vi "car _ai.vi"() -> ()   [LabVIEW 2022 SP3]
uses:
  Control 1.ctl
  Control 2.ctl
  chicken.ctl
  plus_one.ctl
  game_over.ctl
panel:
  in  "v 10":dbl
  in  "v 9":dbl
  in  "v 8":dbl
  in  "v 7":dbl
  in  "v 6":dbl
  in  "v 5":dbl
  in  "v 4":dbl
  in  "v 3":dbl
  in  "v 2":dbl
  in  "v":dbl
  in  "state":i16
  in  "action":i16
  out "Boolean 12":T1
  in  "chicken":T2
  out "TOP":i16
  out "SCORE":i16
  in  "stop":bool
  out "Boolean 11":T3
  out "car_x":i16
  out "Boolean 10":T4
  out "Boolean 9":T5
  out "Boolean 8":T4
  out "Boolean 7":T5
  out "Boolean 6":T4
  out "Boolean 5":T5
  out "Boolean 4":T4
  out "Boolean 3":T5
  out "Boolean 2":T4
  out "Boolean":T5
  # "SCORE"
  # "TOP"
  # "Don't forget to reset the path of music first."
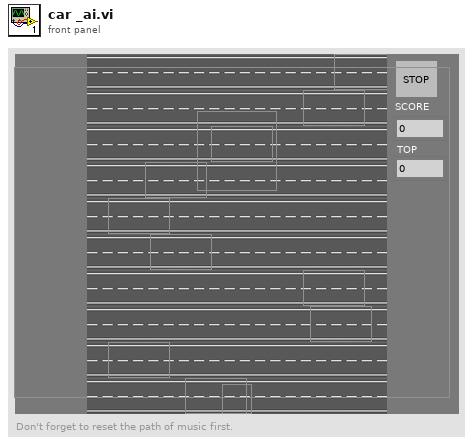
[diagram p1: front panel]
types:
  T1 = typedef "game_over.ctl" = bool
  T2 = typedef "chicken.ctl" = bool
  T3 = typedef "plus_one.ctl" = bool
  T4 = typedef "Control 2.ctl" = bool
  T5 = typedef "Control 1.ctl" = bool
  T6 = typedef "Sound Output Task ID.ctl" = u32
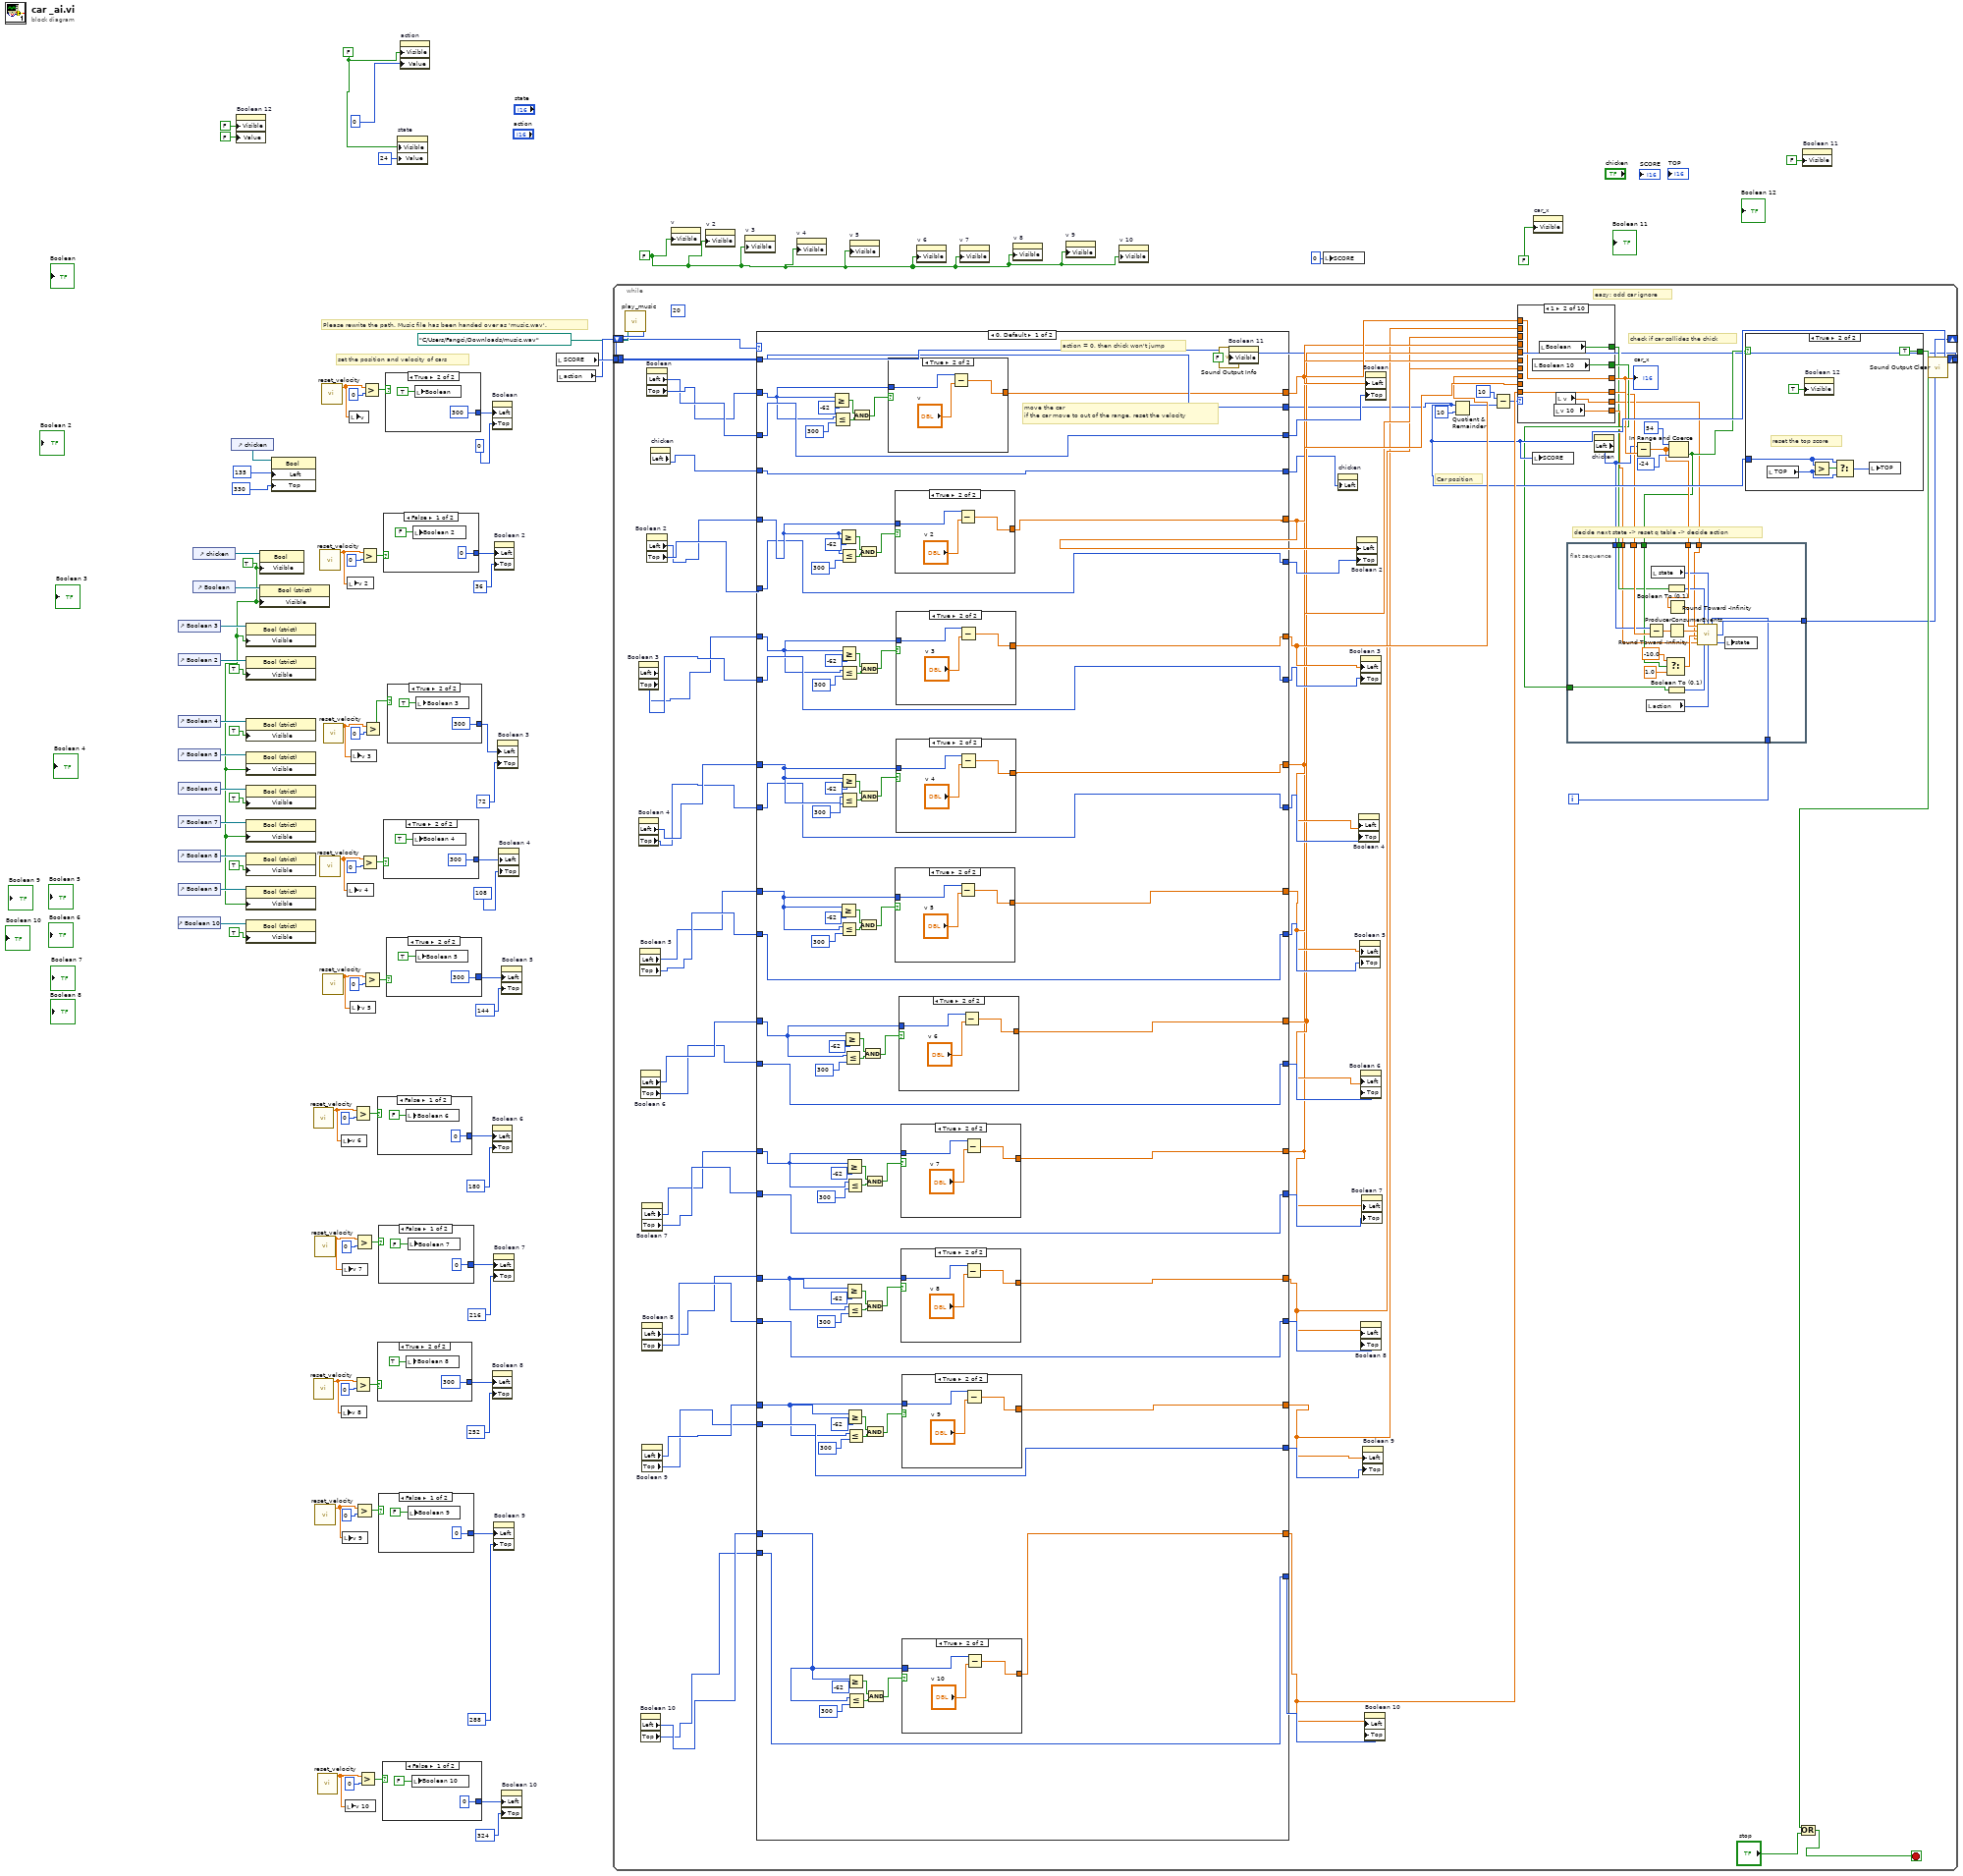
[diagram p0: block diagram]
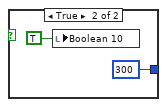
[diagram p2: hidden frame]
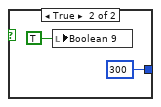
[diagram p3: hidden frame]
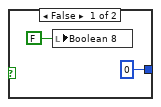
[diagram p4: hidden frame]
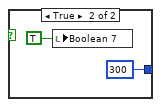
[diagram p5: hidden frame]
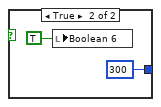
[diagram p6: hidden frame]
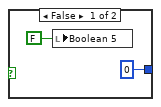
[diagram p7: hidden frame]
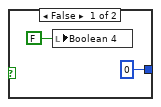
[diagram p8: hidden frame]
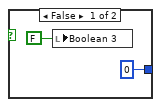
[diagram p9: hidden frame]
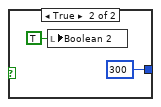
[diagram p10: hidden frame]
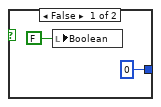
[diagram p11: hidden frame]
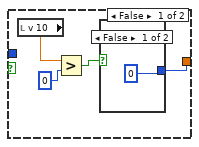
[diagram p12: hidden frame]
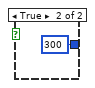
[diagram p13: hidden frame]
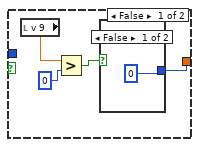
[diagram p14: hidden frame]
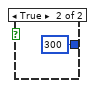
[diagram p15: hidden frame]
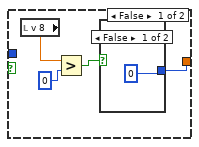
[diagram p16: hidden frame]
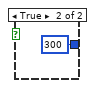
[diagram p17: hidden frame]
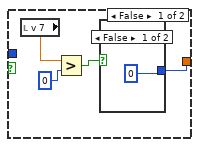
[diagram p18: hidden frame]
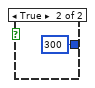
[diagram p19: hidden frame]
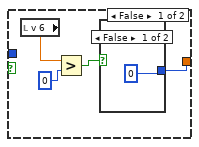
[diagram p20: hidden frame]
diagram:
  w19 = TRUE ("Visible")
  w14 = FALSE ("Visible")
  w17 = FALSE
  # "set the position and velocity of cars"
  # "Please rewrite the path. Music file has been handed over as 'music.wav'."
  n1 = control-ref of="Boolean 3"() -> (w27:refnum<vi>)
  n2 = control-ref of="Boolean 2"() -> (w28:refnum<vi>)
  n3 = control-ref of="Boolean 4"() -> (w29:refnum<vi>)
  n4 = control-ref of="Boolean 5"() -> (w30:refnum<vi>)
  n5 = control-ref of="Boolean 6"() -> (w31:refnum<vi>)
  n6 = control-ref of="Boolean 7"() -> (w32:refnum<vi>)
  n7 = control-ref of="Boolean 8"() -> (w33:refnum<vi>)
  n8 = control-ref of="Boolean 9"() -> (w34:refnum<vi>)
  n9 = control-ref of="Boolean 10"() -> (w36:refnum<vi>)
  n10 = control-ref of="chicken"() -> (w21:refnum<vi>)
  n11 = control-ref of="Boolean"() -> (w26:refnum<vi>)
  n12 = control-ref of="chicken"() -> (w41:refnum<vi>)
  n13 = property on="Boolean 12" class="Bool (strict)"("Visible"=FALSE, "Value"=T1 FALSE ("Boolean 12")) -> ()  [unwired: 2 in, 2 out]
  n14 = property class="Bool (strict)"(reference=w27, "Visible"=w19) -> ()  [unwired: 1 in, 2 out]
  n15 = property class="Bool (strict)"(reference=w28, "Visible"=TRUE) -> ()  [unwired: 1 in, 2 out]
  n16 = property class="Bool (strict)"(reference=w29, "Visible"=TRUE) -> ()  [unwired: 1 in, 2 out]
  n17 = property class="Bool (strict)"(reference=w30, "Visible"=w19) -> ()  [unwired: 1 in, 2 out]
  n18 = property class="Bool (strict)"(reference=w31, "Visible"=TRUE) -> ()  [unwired: 1 in, 2 out]
  n19 = property class="Bool (strict)"(reference=w32, "Visible"=w19) -> ()  [unwired: 1 in, 2 out]
  n20 = property class="Bool (strict)"(reference=w33, "Visible"=TRUE) -> ()  [unwired: 1 in, 2 out]
  n21 = property class="Bool (strict)"(reference=w34, "Visible"=w19) -> ()  [unwired: 1 in, 2 out]
  n22 = property class="Bool (strict)"(reference=w36, "Visible"=TRUE) -> ()  [unwired: 1 in, 2 out]
  n23 = property class="Bool"(reference=w21, "Visible"=w19) -> ()  [unwired: 1 in, 2 out]
  n24 = property class="Bool (strict)"(reference=w26, "Visible"=w19) -> ()  [unwired: 1 in, 2 out]
  n25 = property on="Property Node" class="Bool"(reference=w41, "Left"=135 ("Position:Left"), "Top"=330 ("Position:Top")) -> ()  [unwired: 1 in, 2 out]
  n26 = call "reset_velocity.vi"() -> ("Numeric"=w9:dbl)  [unwired: 11 in]
  n27 = call "reset_velocity.vi"() -> ("Numeric"=w11:dbl)  [unwired: 11 in]
  n28 = call "reset_velocity.vi"() -> ("Numeric"=w10:dbl)  [unwired: 11 in]
  n29 = call "reset_velocity.vi"() -> ("Numeric"=w12:dbl)  [unwired: 11 in]
  n30 = call "reset_velocity.vi"() -> ("Numeric"=w13:dbl)  [unwired: 11 in]
  n31 = call "reset_velocity.vi"() -> ("Numeric"=w5:dbl)  [unwired: 11 in]
  n32 = call "reset_velocity.vi"() -> ("Numeric"=w7:dbl)  [unwired: 11 in]
  n33 = call "reset_velocity.vi"() -> ("Numeric"=w4:dbl)  [unwired: 11 in]
  n34 = call "reset_velocity.vi"() -> ("Numeric"=w8:dbl)  [unwired: 11 in]
  n35 = call "reset_velocity.vi"() -> ("Numeric"=w6:dbl)  [unwired: 11 in]
  n36 = local write "v 6"(w9) -> ()
  n37 = local write "v 8"(w11) -> ()
  n38 = local write "v 7"(w10) -> ()
  n39 = local write "v 9"(w12) -> ()
  n40 = local write "v 10"(w13) -> ()
  n41 = local write "v 2"(w5) -> ()
  n42 = local write "v 4"(w7) -> ()
  n43 = local write "v"(w4) -> ()
  n44 = local write "v 5"(w8) -> ()
  n45 = local write "v 3"(w6) -> ()
  n46 = Greater?(x=w9, y=0) -> (0:w61:bool)
  n47 = Greater?(x=w11, y=0) -> (0:w53:bool)
  n48 = Greater?(x=w10, y=0) -> (0:w56:bool)
  n49 = Greater?(x=w12, y=0) -> (0:w48:bool)
  n50 = Greater?(x=w13, y=0) -> (0:w45:bool)
  n51 = Greater?(x=w5, y=0) -> (0:w77:bool)
  n52 = Greater?(x=w7, y=0) -> (0:w69:bool)
  n53 = Greater?(x=w4, y=0) -> (0:w80:bool)
  n54 = Greater?(x=w8, y=0) -> (0:w64:bool)
  n55 = Greater?(x=w6, y=0) -> (0:w72:bool)
  n56 = case shown="False" w61 {
    tunnel: [0 300] -> w59
    frame False {
      n57 = local write "Boolean 6"(FALSE) -> ()
    }
    frame True {
      n58 = local write "Boolean 6"(TRUE) -> ()
    }
  }
  n59 = case shown="True" w53 {
    tunnel: [0 300] -> w51
    frame False {
      n60 = local write "Boolean 8"(FALSE) -> ()
    }
    frame True {
      n61 = local write "Boolean 8"(TRUE) -> ()
    }
  }
  n62 = case shown="False" w56 {
    tunnel: [0 300] -> w55
    frame False {
      n63 = local write "Boolean 7"(FALSE) -> ()
    }
    frame True {
      n64 = local write "Boolean 7"(TRUE) -> ()
    }
  }
  n65 = case shown="False" w48 {
    tunnel: [0 300] -> w47
    frame False {
      n66 = local write "Boolean 9"(FALSE) -> ()
    }
    frame True {
      n67 = local write "Boolean 9"(TRUE) -> ()
    }
  }
  n68 = case shown="False" w45 {
    tunnel: [0 300] -> w43
    frame False {
      n69 = local write "Boolean 10"(FALSE) -> ()
    }
    frame True {
      n70 = local write "Boolean 10"(TRUE) -> ()
    }
  }
  n71 = case shown="False" w77 {
    tunnel: [0 300] -> w75
    frame False {
      n72 = local write "Boolean 2"(FALSE) -> ()
    }
    frame True {
      n73 = local write "Boolean 2"(TRUE) -> ()
    }
  }
  n74 = case shown="True" w69 {
    tunnel: [0 300] -> w67
    frame False {
      n75 = local write "Boolean 4"(FALSE) -> ()
    }
    frame True {
      n76 = local write "Boolean 4"(TRUE) -> ()
    }
  }
  n77 = case shown="True" w80 {
    tunnel: [0 300] -> w79
    frame False {
      n78 = local write "Boolean"(FALSE) -> ()
    }
    frame True {
      n79 = local write "Boolean"(TRUE) -> ()
    }
  }
  n80 = case shown="True" w64 {
    tunnel: [0 300] -> w63
    frame False {
      n81 = local write "Boolean 5"(FALSE) -> ()
    }
    frame True {
      n82 = local write "Boolean 5"(TRUE) -> ()
    }
  }
  n83 = case shown="True" w72 {
    tunnel: [0 300] -> w70
    frame False {
      n84 = local write "Boolean 3"(FALSE) -> ()
    }
    frame True {
      n85 = local write "Boolean 3"(TRUE) -> ()
    }
  }
  n86 = property on="state" class="DigNum (strict)"("Visible"=w17, "Value"=i16 24 ("state")) -> ()  [unwired: 2 in, 2 out]
  n87 = property on="action" class="DigNum (strict)"("Visible"=w17, "Value"=i16 0 ("done")) -> ()  [unwired: 2 in, 2 out]
  n88 = property on="Boolean" class="Bool (strict)"("Left"=w79, "Top"=0) -> ()  [unwired: 2 in, 2 out]
  n89 = property on="Boolean 6" class="Bool (strict)"("Left"=w59, "Top"=180) -> ()  [unwired: 2 in, 2 out]
  n90 = property on="Boolean 8" class="Bool (strict)"("Left"=w51, "Top"=252) -> ()  [unwired: 2 in, 2 out]
  n91 = property on="Boolean 7" class="Bool (strict)"("Left"=w55, "Top"=216) -> ()  [unwired: 2 in, 2 out]
  n92 = property on="Boolean 9" class="Bool (strict)"("Left"=w47, "Top"=288) -> ()  [unwired: 2 in, 2 out]
  n93 = property on="Boolean 2" class="Bool (strict)"("Left"=w75, "Top"=36) -> ()  [unwired: 2 in, 2 out]
  n94 = property on="Boolean 3" class="Bool (strict)"("Left"=w70, "Top"=72) -> ()  [unwired: 2 in, 2 out]
  n95 = property on="Boolean 4" class="Bool (strict)"("Left"=w67, "Top"=108) -> ()  [unwired: 2 in, 2 out]
  n96 = property on="Boolean 5" class="Bool (strict)"("Left"=w63, "Top"=144) -> ()  [unwired: 2 in, 2 out]
  n97 = property on="Boolean 10" class="Bool (strict)"("Left"=w43, "Top"=324) -> ()  [unwired: 2 in, 2 out]
  n98 = local read "SCORE"() -> (w20:i16)
  n99 = local read "action"() -> (w18:i16)
  n100 = call "play_music.vi"("Sound File Path"=path "C:/Users/Fangci/Downloads/music.wav") -> ("task ID"=w3:T6)  [unwired: 10 in]
  n101 = while {
    shift-right: [w140] -> _
    shift-left: w20 -> [w141]
    shift-right: [w129] -> _
    shift-left: w18 -> [w138]
    tunnel: w3 -> [w126]
    tunnel: [w125] -> w2
    i -> [w128]
    stop <- w127 stop-if-true
    (unwired) 20
    # "decide next state -> reset q table -> decide action"
    # "check if car collides the chick"
    # "easy: odd car ignore"
    # "Car position"
    n102 = property on="Boolean 3" class="Bool (strict)"() -> ("Left"=w184:i32, "Top"=w185:i32)  [unwired: 2 in, 2 out]
    n103 = property on="Boolean 4" class="Bool (strict)"() -> ("Left"=w182:i32, "Top"=w181:i32)  [unwired: 2 in, 2 out]
    n104 = property on="Boolean 5" class="Bool (strict)"() -> ("Left"=w171:i32, "Top"=w179:i32)  [unwired: 2 in, 2 out]
    n105 = property on="Boolean 6" class="Bool (strict)"() -> ("Left"=w177:i32, "Top"=w176:i32)  [unwired: 2 in, 2 out]
    n106 = property on="Boolean 10" class="Bool (strict)"() -> ("Left"=w164:i32, "Top"=w163:i32)  [unwired: 2 in, 2 out]
    n107 = property on="Boolean 7" class="Bool (strict)"() -> ("Left"=w170:i32, "Top"=w174:i32)  [unwired: 2 in, 2 out]
    n108 = property on="Boolean 8" class="Bool (strict)"() -> ("Left"=w169:i32, "Top"=w172:i32)  [unwired: 2 in, 2 out]
    n109 = property on="Boolean 9" class="Bool (strict)"() -> ("Left"=w167:i32, "Top"=w166:i32)  [unwired: 2 in, 2 out]
    n110 = property on="Boolean" class="Bool (strict)"() -> ("Left"=w190:i32, "Top"=w191:i32)  [unwired: 2 in, 2 out]
    n111 = property on="Boolean 2" class="Bool (strict)"() -> ("Left"=w188:i32, "Top"=w189:i32)  [unwired: 2 in, 2 out]
    n112 = property on="chicken" class="Bool"() -> ("Left"=w143:i32)  [unwired: 2 in, 2 out]
    n113 = case shown="0, Default" w138 {
      tunnel: [w223 w426] -> w186
      tunnel: w191 -> [w223 w425]
      tunnel: [w220 w424] -> w160
      tunnel: w190 -> [w222 w423]
      tunnel: [w217 w419] -> w187
      tunnel: w189 -> [w217 w420]
      tunnel: [w216 w421] -> w159
      tunnel: w188 -> [w218 w422]
      tunnel: [w214 w413] -> w183
      tunnel: w185 -> [w214 w414]
      tunnel: [w215 w415] -> w158
      tunnel: w184 -> [w213 w416]
      tunnel: [w211 w408] -> w180
      tunnel: w181 -> [w211 w407]
      tunnel: [w210 w406] -> w157
      tunnel: w182 -> [w212 w405]
      tunnel: [w208 w401] -> w178
      tunnel: w179 -> [w208 w402]
      tunnel: [w209 w403] -> w156
      tunnel: w171 -> [w207 w404]
      tunnel: [w206 w396] -> w175
      tunnel: w176 -> [w206 w395]
      tunnel: [w205 w394] -> w155
      tunnel: w177 -> [w204 w393]
      tunnel: [w202 w389] -> w173
      tunnel: w174 -> [w202 w390]
      tunnel: [w201 w391] -> w154
      tunnel: w170 -> [w203 w392]
      tunnel: [w199 w384] -> w168
      tunnel: w172 -> [w199 w383]
      tunnel: [w198 w382] -> w153
      tunnel: w169 -> [w200 w381]
      tunnel: [w196 w377] -> w165
      tunnel: w166 -> [w196 w378]
      tunnel: [w197 w379] -> w152
      tunnel: w167 -> [w195 w380]
      tunnel: [w192 w372] -> w162
      tunnel: w163 -> [w192 w371]
      tunnel: [w193 w370] -> w151
      tunnel: w164 -> [w194 w369]
      tunnel: w143 -> [w219 w367]
      tunnel: [w219 w367] -> w142
      tunnel: w141 -> [w221 w366]
      tunnel: [w221 w365] -> w140
      frame 0, Default {
        # "move the car\nif the car move to out of the range, reset the velocity"
        # "action = 0, then chick won't jump"
        n114 = Greater Or Equal?(x=w222, y=-62) -> (x >= y?=w246:bool)
        n115 = Less Or Equal?(x=w222, y=300) -> (x <= y?=w245:bool)
        n116 = Greater Or Equal?(x=w218, y=-62) -> (x >= y?=w249:bool)
        n117 = Greater Or Equal?(x=w207, y=-62) -> (x >= y?=w258:bool)
        n118 = Less Or Equal?(x=w218, y=300) -> (x <= y?=w250:bool)
        n119 = Greater Or Equal?(x=w213, y=-62) -> (x >= y?=w252:bool)
        n120 = Greater Or Equal?(x=w212, y=-62) -> (x >= y?=w255:bool)
        n121 = Less Or Equal?(x=w207, y=300) -> (x <= y?=w259:bool)
        n122 = Less Or Equal?(x=w213, y=300) -> (x <= y?=w253:bool)
        n123 = Less Or Equal?(x=w212, y=300) -> (x <= y?=w254:bool)
        n124 = Greater Or Equal?(x=w204, y=-62) -> (x >= y?=w261:bool)
        n125 = Less Or Equal?(x=w204, y=300) -> (x <= y?=w260:bool)
        n126 = Greater Or Equal?(x=w203, y=-62) -> (x >= y?=w264:bool)
        n127 = Greater Or Equal?(x=w200, y=-62) -> (x >= y?=w267:bool)
        n128 = Less Or Equal?(x=w203, y=300) -> (x <= y?=w265:bool)
        n129 = Less Or Equal?(x=w200, y=300) -> (x <= y?=w266:bool)
        n130 = Greater Or Equal?(x=w195, y=-62) -> (x >= y?=w270:bool)
        n131 = Less Or Equal?(x=w195, y=300) -> (x <= y?=w271:bool)
        n132 = Greater Or Equal?(x=w194, y=-62) -> (x >= y?=w273:bool)
        n133 = Less Or Equal?(x=w194, y=300) -> (x <= y?=w272:bool)
        n134 = And(x=w246, y=w245) -> (x .and. y?=w247:bool)
        n135 = And(x=w249, y=w250) -> (x .and. y?=w248:bool)
        n136 = And(x=w258, y=w259) -> (x .and. y?=w257:bool)
        n137 = And(x=w252, y=w253) -> (x .and. y?=w251:bool)
        n138 = And(x=w255, y=w254) -> (x .and. y?=w256:bool)
        n139 = And(x=w261, y=w260) -> (x .and. y?=w262:bool)
        n140 = And(x=w264, y=w265) -> (x .and. y?=w263:bool)
        n141 = And(x=w267, y=w266) -> (x .and. y?=w268:bool)
        n142 = And(x=w270, y=w271) -> (x .and. y?=w269:bool)
        n143 = And(x=w273, y=w272) -> (x .and. y?=w274:bool)
        n144 = case shown="True" w247 {
          tunnel: [w356 w363] -> w220
          tunnel: w222 -> [_ w362]
          frame False {
            n145 = local read "v"() -> (w359:dbl)
            n146 = Greater?(x=w359, y=0) -> (0:w357:bool)
            n147 = case shown="False" w357 {
              tunnel: [0 300] -> w356
              frame False {
              }
              frame True {
              }
            }
          }
          frame True {
            n148 = Subtract(x=w362, y="v") -> (x-y=w363:dbl)
          }
        }
        n149 = case shown="True" w248 {
          tunnel: [w347 w354] -> w216
          tunnel: w218 -> [_ w353]
          frame False {
            n150 = local read "v 2"() -> (w350:dbl)
            n151 = Greater?(x=w350, y=0) -> (0:w348:bool)
            n152 = case shown="False" w348 {
              tunnel: [0 300] -> w347
              frame False {
              }
              frame True {
              }
            }
          }
          frame True {
            n153 = Subtract(x=w353, y="v 2") -> (x-y=w354:dbl)
          }
        }
        n154 = case shown="True" w257 {
          tunnel: [w320 w327] -> w209
          tunnel: w207 -> [_ w326]
          frame False {
            n155 = local read "v 5"() -> (w323:dbl)
            n156 = Greater?(x=w323, y=0) -> (0:w321:bool)
            n157 = case shown="False" w321 {
              tunnel: [0 300] -> w320
              frame False {
              }
              frame True {
              }
            }
          }
          frame True {
            n158 = Subtract(x=w326, y="v 5") -> (x-y=w327:dbl)
          }
        }
        n159 = case shown="True" w251 {
          tunnel: [w338 w345] -> w215
          tunnel: w213 -> [_ w344]
          frame False {
            n160 = local read "v 3"() -> (w341:dbl)
            n161 = Greater?(x=w341, y=0) -> (0:w339:bool)
            n162 = case shown="False" w339 {
              tunnel: [0 300] -> w338
              frame False {
              }
              frame True {
              }
            }
          }
          frame True {
            n163 = Subtract(x=w344, y="v 3") -> (x-y=w345:dbl)
          }
        }
        n164 = case shown="True" w256 {
          tunnel: [w329 w336] -> w210
          tunnel: w212 -> [_ w335]
          frame False {
            n165 = local read "v 4"() -> (w332:dbl)
            n166 = Greater?(x=w332, y=0) -> (0:w330:bool)
            n167 = case shown="False" w330 {
              tunnel: [0 300] -> w329
              frame False {
              }
              frame True {
              }
            }
          }
          frame True {
            n168 = Subtract(x=w335, y="v 4") -> (x-y=w336:dbl)
          }
        }
        n169 = case shown="True" w262 {
          tunnel: [w311 w318] -> w205
          tunnel: w204 -> [_ w317]
          frame False {
            n170 = local read "v 6"() -> (w314:dbl)
            n171 = Greater?(x=w314, y=0) -> (0:w312:bool)
            n172 = case shown="False" w312 {
              tunnel: [0 300] -> w311
              frame False {
              }
              frame True {
              }
            }
          }
          frame True {
            n173 = Subtract(x=w317, y="v 6") -> (x-y=w318:dbl)
          }
        }
        n174 = case shown="True" w263 {
          tunnel: [w302 w309] -> w201
          tunnel: w203 -> [_ w308]
          frame False {
            n175 = local read "v 7"() -> (w305:dbl)
            n176 = Greater?(x=w305, y=0) -> (0:w303:bool)
            n177 = case shown="False" w303 {
              tunnel: [0 300] -> w302
              frame False {
              }
              frame True {
              }
            }
          }
          frame True {
            n178 = Subtract(x=w308, y="v 7") -> (x-y=w309:dbl)
          }
        }
        n179 = case shown="True" w268 {
          tunnel: [w293 w300] -> w198
          tunnel: w200 -> [_ w299]
          frame False {
            n180 = local read "v 8"() -> (w296:dbl)
            n181 = Greater?(x=w296, y=0) -> (0:w294:bool)
            n182 = case shown="False" w294 {
              tunnel: [0 300] -> w293
              frame False {
              }
              frame True {
              }
            }
          }
          frame True {
            n183 = Subtract(x=w299, y="v 8") -> (x-y=w300:dbl)
          }
        }
        n184 = case shown="True" w269 {
          tunnel: [w284 w291] -> w197
          tunnel: w195 -> [_ w290]
          frame False {
            n185 = local read "v 9"() -> (w287:dbl)
            n186 = Greater?(x=w287, y=0) -> (0:w285:bool)
            n187 = case shown="False" w285 {
              tunnel: [0 300] -> w284
              frame False {
              }
              frame True {
              }
            }
          }
          frame True {
            n188 = Subtract(x=w290, y="v 9") -> (x-y=w291:dbl)
          }
        }
        n189 = case shown="True" w274 {
          tunnel: [w275 w282] -> w193
          tunnel: w194 -> [_ w281]
          frame False {
            n190 = local read "v 10"() -> (w278:dbl)
            n191 = Greater?(x=w278, y=0) -> (0:w276:bool)
            n192 = case shown="False" w276 {
              tunnel: [0 300] -> w275
              frame False {
              }
              frame True {
              }
            }
          }
          frame True {
            n193 = Subtract(x=w281, y="v 10") -> (x-y=w282:dbl)
          }
        }
        n194 = property on="Boolean 11" class="Bool (strict)"("Visible"=FALSE) -> ()  [unwired: 2 in, 2 out]
      }
      frame 1 {
        # "move the car\nif the car move to out of the range, reset the velocity"
        # "action = 1, then chick  jumps"
        n195 = Less?(x=w420, y=324) -> (x < y?=w417:bool)
        n196 = Less?(x=w383, y=324) -> (x < y?=w386:bool)
        n197 = Less?(x=w414, y=324) -> (x < y?=w411:bool)
        n198 = Less?(x=w390, y=324) -> (x < y?=w387:bool)
        n199 = Less?(x=w371, y=324) -> (x < y?=w374:bool)
        n200 = Less?(x=w407, y=324) -> (x < y?=w410:bool)
        n201 = Less?(x=w402, y=324) -> (x < y?=w399:bool)
        n202 = Less?(x=w395, y=324) -> (x < y?=w398:bool)
        n203 = Less?(x=w378, y=324) -> (x < y?=w375:bool)
        n204 = Less?(x=w425, y=324) -> (x < y?=w428:bool)
        n205 = case shown="False" w417 {
          tunnel: [0 w563] -> w419
          tunnel: w420 -> [_ w562]
          tunnel: [w550 w560] -> w421
          tunnel: w422 -> [_ w559]
          frame False {
            n206 = call "reset_velocity.vi"() -> ("Numeric"=w549:dbl)  [unwired: 11 in]
            n207 = local write "v 2"(w549) -> ()
            n208 = Greater?(x=w549, y=0) -> (0:w554:bool)
            n209 = case shown="False" w554 {
              frame False {
                n210 = local write "Boolean 2"(FALSE) -> ()
              }
              frame True {
                n211 = local write "Boolean 2"(TRUE) -> ()
              }
            }
            n212 = Random Number (0-1)() -> (number: 0 to 1=w552:dbl)
            n213 = Multiply(x=w552, y=300) -> (x*y=w550:dbl)
          }
          frame True {
            n214 = Add(x=w562, y=36) -> (x+y=w563:i32)
            n215 = local read "v 2"() -> (w558:dbl)
            n216 = Subtract(x=w559, y=w558) -> (x-y=w560:dbl)
          }
        }
        n217 = case shown="False" w386 {
          tunnel: [0 w473] -> w384
          tunnel: w383 -> [_ w472]
          tunnel: [w460 w469] -> w382
          tunnel: w381 -> [_ w470]
          frame False {
            n218 = call "reset_velocity.vi"() -> ("Numeric"=w459:dbl)  [unwired: 11 in]
            n219 = local write "v 8"(w459) -> ()
            n220 = Greater?(x=w459, y=0) -> (0:w464:bool)
            n221 = case shown="False" w464 {
              frame False {
                n222 = local write "Boolean 8"(FALSE) -> ()
              }
              frame True {
                (unwired) 300
                n223 = local write "Boolean 8"(TRUE) -> ()
              }
            }
            n224 = Random Number (0-1)() -> (number: 0 to 1=w461:dbl)
            n225 = Multiply(x=w461, y=300) -> (x*y=w460:dbl)
          }
          frame True {
            n226 = Add(x=w472, y=36) -> (x+y=w473:i32)
            n227 = local read "v 8"() -> (w468:dbl)
            n228 = Subtract(x=w470, y=w468) -> (x-y=w469:dbl)
          }
        }
        n229 = case shown="False" w411 {
          tunnel: [0 w548] -> w413
          tunnel: w414 -> [_ w547]
          tunnel: [w535 w544] -> w415
          tunnel: w416 -> [_ w545]
          frame False {
            n230 = call "reset_velocity.vi"() -> ("Numeric"=w534:dbl)  [unwired: 11 in]
            n231 = local write "v 3"(w534) -> ()
            n232 = Greater?(x=w534, y=0) -> (0:w539:bool)
            n233 = case shown="True" w539 {
              frame False {
                (unwired) 0
                n234 = local write "Boolean 3"(FALSE) -> ()
              }
              frame True {
                n235 = local write "Boolean 3"(TRUE) -> ()
              }
            }
            n236 = Random Number (0-1)() -> (number: 0 to 1=w537:dbl)
            n237 = Multiply(x=w537, y=300) -> (x*y=w535:dbl)
          }
          frame True {
            n238 = Add(x=w547, y=36) -> (x+y=w548:i32)
            n239 = local read "v 3"() -> (w543:dbl)
            n240 = Subtract(x=w545, y=w543) -> (x-y=w544:dbl)
          }
        }
        n241 = case shown="False" w387 {
          tunnel: [0 w488] -> w389
          tunnel: w390 -> [_ w487]
          tunnel: [w475 w484] -> w391
          tunnel: w392 -> [_ w485]
          frame False {
            n242 = call "reset_velocity.vi"() -> ("Numeric"=w474:dbl)  [unwired: 11 in]
            n243 = local write "v 7"(w474) -> ()
            n244 = Greater?(x=w474, y=0) -> (0:w479:bool)
            n245 = case shown="True" w479 {
              frame False {
                (unwired) 0
                n246 = local write "Boolean 7"(FALSE) -> ()
              }
              frame True {
                n247 = local write "Boolean 7"(TRUE) -> ()
              }
            }
            n248 = Random Number (0-1)() -> (number: 0 to 1=w477:dbl)
            n249 = Multiply(x=w477, y=300) -> (x*y=w475:dbl)
          }
          frame True {
            n250 = local read "v 7"() -> (w483:dbl)
            n251 = Add(x=w487, y=36) -> (x+y=w488:i32)
            n252 = Subtract(x=w485, y=w483) -> (x-y=w484:dbl)
          }
        }
        n253 = case shown="False" w374 {
          tunnel: [0 w443] -> w372
          tunnel: w371 -> [_ w442]
          tunnel: [w430 w439] -> w370
          tunnel: w369 -> [_ w440]
          frame False {
            n254 = call "reset_velocity.vi"() -> ("Numeric"=w429:dbl)  [unwired: 11 in]
            n255 = local write "v 10"(w429) -> ()
            n256 = Greater?(x=w429, y=0) -> (0:w434:bool)
            n257 = case shown="False" w434 {
              frame False {
                n258 = local write "Boolean 10"(FALSE) -> ()
              }
              frame True {
                (unwired) 300
                n259 = local write "Boolean 10"(TRUE) -> ()
              }
            }
            n260 = Random Number (0-1)() -> (number: 0 to 1=w431:dbl)
            n261 = Multiply(x=w431, y=300) -> (x*y=w430:dbl)
          }
          frame True {
            n262 = Add(x=w442, y=36) -> (x+y=w443:i32)
            n263 = local read "v 10"() -> (w438:dbl)
            n264 = Subtract(x=w440, y=w438) -> (x-y=w439:dbl)
          }
        }
        n265 = case shown="False" w410 {
          tunnel: [0 w533] -> w408
          tunnel: w407 -> [_ w532]
          tunnel: [w520 w529] -> w406
          tunnel: w405 -> [_ w530]
          frame False {
            n266 = call "reset_velocity.vi"() -> ("Numeric"=w519:dbl)  [unwired: 11 in]
            n267 = local write "v 4"(w519) -> ()
            n268 = Greater?(x=w519, y=0) -> (0:w524:bool)
            n269 = case shown="False" w524 {
              frame False {
                n270 = local write "Boolean 4"(FALSE) -> ()
              }
              frame True {
                (unwired) 300
                n271 = local write "Boolean 4"(TRUE) -> ()
              }
            }
            n272 = Random Number (0-1)() -> (number: 0 to 1=w522:dbl)
            n273 = Multiply(x=w522, y=300) -> (x*y=w520:dbl)
          }
          frame True {
            n274 = Add(x=w532, y=36) -> (x+y=w533:i32)
            n275 = local read "v 4"() -> (w528:dbl)
            n276 = Subtract(x=w530, y=w528) -> (x-y=w529:dbl)
          }
        }
        n277 = case shown="False" w399 {
          tunnel: [0 w518] -> w401
          tunnel: w402 -> [_ w517]
          tunnel: [w505 w514] -> w403
          tunnel: w404 -> [_ w515]
          frame False {
            n278 = call "reset_velocity.vi"() -> ("Numeric"=w504:dbl)  [unwired: 11 in]
            n279 = local write "v 5"(w504) -> ()
            n280 = Greater?(x=w504, y=0) -> (0:w509:bool)
            n281 = case shown="True" w509 {
              frame False {
                (unwired) 0
                n282 = local write "Boolean 5"(FALSE) -> ()
              }
              frame True {
                n283 = local write "Boolean 5"(TRUE) -> ()
              }
            }
            n284 = Random Number (0-1)() -> (number: 0 to 1=w506:dbl)
            n285 = Multiply(x=w506, y=300) -> (x*y=w505:dbl)
          }
          frame True {
            n286 = local read "v 5"() -> (w513:dbl)
            n287 = Add(x=w517, y=36) -> (x+y=w518:i32)
            n288 = Subtract(x=w515, y=w513) -> (x-y=w514:dbl)
          }
        }
        n289 = case shown="False" w398 {
          tunnel: [0 w503] -> w396
          tunnel: w395 -> [_ w502]
          tunnel: [w490 w499] -> w394
          tunnel: w393 -> [_ w500]
          frame False {
            n290 = call "reset_velocity.vi"() -> ("Numeric"=w489:dbl)  [unwired: 11 in]
            n291 = local write "v 6"(w489) -> ()
            n292 = Greater?(x=w489, y=0) -> (0:w494:bool)
            n293 = case shown="False" w494 {
              frame False {
                n294 = local write "Boolean 6"(FALSE) -> ()
              }
              frame True {
                (unwired) 300
                n295 = local write "Boolean 6"(TRUE) -> ()
              }
            }
            n296 = Random Number (0-1)() -> (number: 0 to 1=w492:dbl)
            n297 = Multiply(x=w492, y=300) -> (x*y=w490:dbl)
          }
          frame True {
            n298 = Add(x=w502, y=36) -> (x+y=w503:i32)
            n299 = local read "v 6"() -> (w498:dbl)
            n300 = Subtract(x=w500, y=w498) -> (x-y=w499:dbl)
          }
        }
        n301 = case shown="False" w375 {
          tunnel: [0 w458] -> w377
          tunnel: w378 -> [_ w457]
          tunnel: [w445 w454] -> w379
          tunnel: w380 -> [_ w455]
          frame False {
            n302 = call "reset_velocity.vi"() -> ("Numeric"=w444:dbl)  [unwired: 11 in]
            n303 = local write "v 9"(w444) -> ()
            n304 = Greater?(x=w444, y=0) -> (0:w449:bool)
            n305 = case shown="True" w449 {
              frame False {
                (unwired) 0
                n306 = local write "Boolean 9"(FALSE) -> ()
              }
              frame True {
                n307 = local write "Boolean 9"(TRUE) -> ()
              }
            }
            n308 = Random Number (0-1)() -> (number: 0 to 1=w447:dbl)
            n309 = Multiply(x=w447, y=300) -> (x*y=w445:dbl)
          }
          frame True {
            n310 = Add(x=w457, y=36) -> (x+y=w458:i32)
            n311 = local read "v 9"() -> (w453:dbl)
            n312 = Subtract(x=w455, y=w453) -> (x-y=w454:dbl)
          }
        }
        n313 = case shown="False" w428 {
          tunnel: [0 w578] -> w426
          tunnel: w425 -> [_ w577]
          tunnel: [w565 w574] -> w424
          tunnel: w423 -> [_ w575]
          frame False {
            n314 = call "reset_velocity.vi"() -> ("Numeric"=w564:dbl)  [unwired: 11 in]
            n315 = local write "v"(w564) -> ()
            n316 = Greater?(x=w564, y=0) -> (0:w569:bool)
            n317 = case shown="False" w569 {
              frame False {
                n318 = local write "Boolean"(FALSE) -> ()
              }
              frame True {
                n319 = local write "Boolean"(TRUE) -> ()
              }
            }
            n320 = Random Number (0-1)() -> (number: 0 to 1=w567:dbl)
            n321 = Multiply(x=w567, y=300) -> (x*y=w565:dbl)
          }
          frame True {
            n322 = Add(x=w577, y=36) -> (x+y=w578:i32)
            n323 = local read "v"() -> (w573:dbl)
            n324 = Subtract(x=w575, y=w573) -> (x-y=w574:dbl)
          }
        }
        n325 = Increment(x=w366) -> (x+1=w365:i16)
        n326 = property on="Boolean 11" class="Bool (strict)"("Visible"=TRUE) -> ()  [unwired: 2 in, 2 out]
      }
    }
    n327 = call <vilib>:"Sound Output Info.vi"("task ID"=w126) -> ("task ID out"=w125:T6)  [unwired: 7 in, 3 out]
    n328 = property on="chicken" class="Bool"("Left"=w142) -> ()  [unwired: 2 in, 2 out]
    n329 = property on="Boolean 2" class="Bool (strict)"("Left"=w159, "Top"=w187) -> ()  [unwired: 2 in, 2 out]
    n330 = property on="Boolean 4" class="Bool (strict)"("Left"=w157, "Top"=w180) -> ()  [unwired: 2 in, 2 out]
    n331 = property on="Boolean 5" class="Bool (strict)"("Left"=w156, "Top"=w178) -> ()  [unwired: 2 in, 2 out]
    n332 = property on="Boolean 3" class="Bool (strict)"("Left"=w158, "Top"=w183) -> ()  [unwired: 2 in, 2 out]
    n333 = property on="Boolean 6" class="Bool (strict)"("Left"=w155, "Top"=w175) -> ()  [unwired: 2 in, 2 out]
    n334 = property on="Boolean 8" class="Bool (strict)"("Left"=w153, "Top"=w168) -> ()  [unwired: 2 in, 2 out]
    n335 = property on="Boolean 7" class="Bool (strict)"("Left"=w154, "Top"=w173) -> ()  [unwired: 2 in, 2 out]
    n336 = property on="Boolean 9" class="Bool (strict)"("Left"=w152, "Top"=w165) -> ()  [unwired: 2 in, 2 out]
    n337 = property on="Boolean 10" class="Bool (strict)"("Left"=w151, "Top"=w162) -> ()  [unwired: 2 in, 2 out]
    n338 = property on="Boolean" class="Bool (strict)"("Left"=w160, "Top"=w186) -> ()  [unwired: 2 in, 2 out]
    n339 = Quotient & Remainder(x=w140, y=i16 10) -> (x-y*floor(x/y)=w148:i16)  [unwired: 1 out]
    n340 = Subtract(x=i16 10, y=w148) -> (x-y=w144:i16)
    n341 = case shown="1" w144 {
      tunnel: w160 -> [_ w618 w621 _ _ _ _ _ _ _]
      tunnel: w159 -> [_ _ w624 w627 _ _ _ _ _ _]
      tunnel: w158 -> [_ _ _ w630 w631 _ _ _ _ _]
      tunnel: w157 -> [_ _ _ _ w636 w639 _ _ _ _]
      tunnel: w156 -> [_ _ _ _ _ w642 w645 _ _ _]
      tunnel: w155 -> [_ _ _ _ _ _ w648 w653 _ _]
      tunnel: w154 -> [_ _ _ _ _ _ _ w654 w659 _]
      tunnel: w153 -> [_ _ _ _ _ _ _ _ w660 w665]
      tunnel: w152 -> [w611 _ _ _ _ _ _ _ _ w666]
      tunnel: w151 -> [w612 w615 _ _ _ _ _ _ _ _]
      tunnel: [w612 w618 w624 w630 w636 w642 w648 w654 w660 w666] -> w139
      tunnel: [w610 w617 w623 w629 w635 w641 w647 w652 w656 w664] -> w130
      tunnel: [w609 w616 w622 w628 w634 w640 w646 w651 w655 w663] -> w137
      tunnel: [w608 w614 w620 w626 w633 w638 w644 w650 w658 w662] -> w132
      tunnel: [w607 w613 w619 w625 w632 w637 w643 w649 w657 w661] -> w131
      tunnel: [w611 w615 w621 w627 w631 w639 w645 w653 w659 w665] -> w135
      frame 10, Default {
        n342 = local read "Boolean 10"() -> (w610:T4)
        n343 = local read "v 10"() -> (w608:dbl)
        n344 = local read "Boolean 9"() -> (w609:T5)
        n345 = local read "v 9"() -> (w607:dbl)
      }
      frame 1 {
        n346 = local read "Boolean 10"() -> (w616:T4)
        n347 = local read "Boolean"() -> (w617:T5)
        n348 = local read "v 10"() -> (w613:dbl)
        n349 = local read "v"() -> (w614:dbl)
      }
      frame 2 {
        n350 = local read "v"() -> (w619:dbl)
        n351 = local read "Boolean 2"() -> (w623:T4)
        n352 = local read "Boolean"() -> (w622:T5)
        n353 = local read "v 2"() -> (w620:dbl)
      }
      frame 3 {
        n354 = local read "v 2"() -> (w625:dbl)
        n355 = local read "Boolean 3"() -> (w629:T5)
        n356 = local read "Boolean 2"() -> (w628:T4)
        n357 = local read "v 3"() -> (w626:dbl)
      }
      frame 4 {
        n358 = local read "Boolean 4"() -> (w635:T4)
        n359 = local read "Boolean 3"() -> (w634:T5)
        n360 = local read "v 3"() -> (w632:dbl)
        n361 = local read "v 4"() -> (w633:dbl)
      }
      frame 5 {
        n362 = local read "Boolean 5"() -> (w641:T5)
        n363 = local read "Boolean 4"() -> (w640:T4)
        n364 = local read "v 5"() -> (w638:dbl)
        n365 = local read "v 4"() -> (w637:dbl)
      }
      frame 6 {
        n366 = local read "Boolean 5"() -> (w646:T5)
        n367 = local read "Boolean 6"() -> (w647:T4)
        n368 = local read "v 6"() -> (w644:dbl)
        n369 = local read "v 5"() -> (w643:dbl)
      }
      frame 7 {
        n370 = local read "Boolean 6"() -> (w651:T4)
        n371 = local read "Boolean 7"() -> (w652:T5)
        n372 = local read "v 6"() -> (w649:dbl)
        n373 = local read "v 7"() -> (w650:dbl)
      }
      frame 8 {
        n374 = local read "Boolean 7"() -> (w655:T5)
        n375 = local read "Boolean 8"() -> (w656:T4)
        n376 = local read "v 7"() -> (w657:dbl)
        n377 = local read "v 8"() -> (w658:dbl)
      }
      frame 9 {
        n378 = local read "Boolean 9"() -> (w664:T5)
        n379 = local read "v 8"() -> (w661:dbl)
        n380 = local read "v 9"() -> (w662:dbl)
        n381 = local read "Boolean 8"() -> (w663:T4)
      }
    }
    "car_x" <- w139
    n382 = local write "SCORE"(w140) -> ()
    n383 = flat-sequence {
      tunnel: w137 -> [w599]
      tunnel: w136 -> [w598]
      tunnel: w135 -> [w597]
      tunnel: w134 -> [w596]
      tunnel: w133 -> [w592]
      tunnel: w132 -> [w580]
      tunnel: w131 -> [w581]
      tunnel: w130 -> [w588]
      tunnel: w128 -> [w579]
      tunnel: [w583] -> w129
      frame #0 {
        n384 = Subtract(x=w596, y=w597) -> (x-y=w595:dbl)
        n385 = local read "action"() -> (w585:i16)
        n386 = local read "state"() -> (w584:i16)
        n387 = Select(t=-10.0, s=w592, f=1.0) -> (s? t:f=w589:dbl)
        n388 = Boolean To (0,1)(Boolean=w588) -> (0, 1=w587:i16)
        n389 = Boolean To (0,1)(Boolean=w599) -> (0, 1=w586:i16)
        n390 = Round Toward -Infinity(1:w595) -> (0:w593:dbl)
        n391 = Round Toward -Infinity(1:w598) -> (0:w594:dbl)
        n392 = call "ProducerConsumerEvents.vi"("d1"=w594, "from_right1"=w587, "state"=w584, "Numeric"=w579, "d2"=w593, "reward"=w589, "v1"=w580, "v2"=w581, "frome_right2"=w586, "ori_action"=w585) -> ("action"=w583:i16, "new_state"=w582:i16)  [unwired: 4 in]
        n393 = local write "state"(w582) -> ()
      }
    }
    n394 = property on="chicken" class="Bool"() -> ("Left"=w134:i32)  [unwired: 2 in, 2 out]
    n395 = Subtract(x=w134, y=w139) -> (x-y=w136:dbl)
    n396 = In Range and Coerce(upper limit=i16 54 ("lower limit"), x=w136, lower limit=i16 -24) -> (In Range?=w133:bool)  [unwired: 1 out]
    n397 = case shown="True" w133 {
      tunnel: w140 -> [_ w604]
      tunnel: [FALSE TRUE] -> w149
      frame False {
      }
      frame True {
        # "reset the top score"
        n398 = local read "TOP"() -> (w605:i16)
        n399 = property on="Boolean 12" class="Bool (strict)"("Visible"=TRUE) -> ()  [unwired: 2 in, 2 out]
        n400 = Greater?(x=w604, y=w605) -> (0:w606:bool)
        n401 = Select(t=w604, s=w606, f=w605) -> (s? t:f=w603:i16)
        n402 = local write "TOP"(w603) -> ()
      }
    }
    n403 = Or(x=w149, y="stop") -> (x .or. y?=w127:bool)
  }
  n404 = property on="v" class="DigNum (strict)"("Visible"=w14) -> ()  [unwired: 2 in, 2 out]
  n405 = property on="v 2" class="DigNum (strict)"("Visible"=w14) -> ()  [unwired: 2 in, 2 out]
  n406 = property on="v 3" class="DigNum (strict)"("Visible"=w14) -> ()  [unwired: 2 in, 2 out]
  n407 = property on="v 4" class="DigNum (strict)"("Visible"=w14) -> ()  [unwired: 2 in, 2 out]
  n408 = property on="v 5" class="DigNum (strict)"("Visible"=w14) -> ()  [unwired: 2 in, 2 out]
  n409 = property on="v 6" class="DigNum (strict)"("Visible"=w14) -> ()  [unwired: 2 in, 2 out]
  n410 = property on="v 7" class="DigNum (strict)"("Visible"=w14) -> ()  [unwired: 2 in, 2 out]
  n411 = property on="v 8" class="DigNum (strict)"("Visible"=w14) -> ()  [unwired: 2 in, 2 out]
  n412 = property on="v 9" class="DigNum (strict)"("Visible"=w14) -> ()  [unwired: 2 in, 2 out]
  n413 = property on="v 10" class="DigNum (strict)"("Visible"=w14) -> ()  [unwired: 2 in, 2 out]
  n414 = local write "SCORE"(i16 0 ("score")) -> ()
  n415 = property on="car_x" class="DigNum (strict)"("Visible"=FALSE) -> ()  [unwired: 2 in, 2 out]
  n416 = property on="Boolean 11" class="Bool (strict)"("Visible"=FALSE) -> ()  [unwired: 2 in, 2 out]
  n417 = call <vilib>:"Sound Output Clear.vi"("task ID"=w2) -> ()  [unwired: 10 in, 1 out]
